vi "RSZVB Set Reference Frequency.vi"(8 "error in (no error)":errorcluster {"code" format="%.0x"}, 11 "VISA session":refnum<visa-resource-name>) -> (0 "error out":errorcluster {"code" format="%.0x"}, 3 "dup VISA session":refnum<visa-resource-name>)   [LabVIEW 2011]
doc: "This VI specifies the frequency of the external reference oscillator.\n\nNote(s):\n\n(1) The frequency must be 10 MHz.\n\nRemote-control command(s):\n[SENSe<Ch>:]ROSCillator:EXTernal:FREQuency 10000000.0"
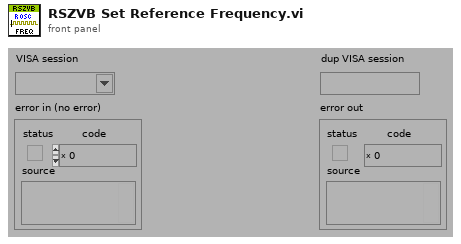
[diagram p1: front panel]
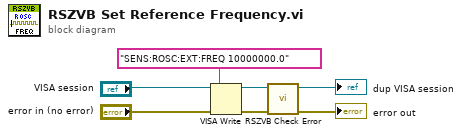
[diagram p0: block diagram]
diagram:
  n1 = VISA Write(VISA resource name="VISA session", write buffer="SENS:ROSC:EXT:FREQ 10000000.0", error in (no error)="error in (no error)") -> (VISA resource name out=w6:refnum<visa-resource-name>, error out=w7:errorcluster)  [unwired: 1 out]
  n2 = call "RSZVB Check Error.vi"("error in (no error)"=w7, "VISA session"=w6) -> ("error out"=→"error out":errorcluster, "dup VISA session"=→"dup VISA session":refnum<visa-resource-name>)  [unwired: 8 in]
